vi "Override To Nominal State.vi"(11 "Base Actor in":refnum<class "Base Actor.lvclass">) -> (3 "Base Actor out":refnum<class "Base Actor.lvclass">)   [LabVIEW 2021, in "jettl.lvlib" / "Actor.lvlib" / "Base Actor.lvclass"]
uses:
  Base Actor.lvclass
  State.ctl
  Base Actor.lvclass/Base Actor.ctl
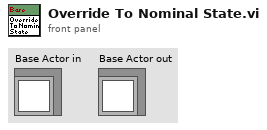
[diagram p1: front panel]
types:
  T1 = typedef "jettl.lvlib/Actor.lvlib/Base Actor.lvclass/State.ctl" = enum16{"Nominal", "Teardown", "Error"}
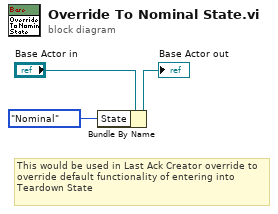
[diagram p0: block diagram]
diagram:
  # "This would be used in Last Ack Creator override to override default functionality of entering into Teardown State"
  n1 = Bundle By Name(cluster="Base Actor in", "State"=State."Nominal") -> (→"Base Actor out":refnum<class "Base Actor.lvclass">)
